vi "Data_Save_GRR.vi"(11 "Data in":T1) -> (1 "Erroe":string[](array[string]), 3 "GRRData":string[](array[string]))   [LabVIEW 2017]
uses:
  Ctrls/CSV_Data.ctl
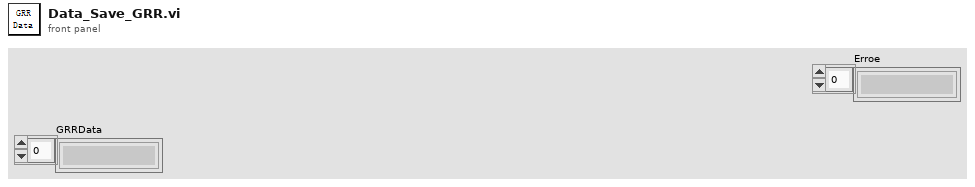
[diagram p1: front panel]
types:
  T1 = typedef "CSV_Data.ctl" = cluster{"Initialisation":cluster{"LMT - Connect UUT (con COM)":string, "LMT - Software Version (rrel)":string, "LMT - Write SKU file (wskuc)":string, "LMT - SKU file name":string, "Connect UUT DDM":string, "Read DDM EOL Timestamp - Mode":string, "Read DDM EOL Timestamp - Timestamp":string, "Read DDM EOL Timestamp - Rig ID":string, "Read DDM EOL Timestamp - Passmark ID":string, "Read DDM EOL Timestamp - Passmark Rev":string, "Software Version before flashing":string, "Read Hardware Serial":string, "UUT DDM SN":string, "Compare DDM SN with MES SN":string, "Backup PCBA Calibration EEPROM Response - CAL":string, "Flash Firmware Version":string, "Check SW Version":string, "Read DDM SW Version after flashing":string, "Set SKU Config":string, "Ready Status":string, "Set Device Mode to EOL":string, "DDM Parameter - Voltage":string, "DDM Parameter - Current":string, "DDM Parameter - Power":string, "DDM Parameter - Speed":string, "DDM Parameter - Pressure":string, "Tester Parameter - Voltage":string, "Tester Parameter - Current":string, "Tester Parameter - Power":string, "Tester Parameter - Ambient Pressure":string, "Tester Parameter - Ambient Temperature":string, "Calculated Parameter - DDM Pressure Corrected":string, "Calculated Parameter - DDM Real Power":string, "Calculated Parameter - Delta V":string}, "BEMF_Calibration":cluster{"Calibration Result - eol_cold_bemf_temp":string, "DDM Ambient Temp":string, "Restriction Plate Diameter":string, "Calibration Result - eol_bemf_mp_cold_coef_a":string, "Calibration Result - eol_bemf_mp_cold_coef_b":string, "Calibration Result - eol_bemf_mp_cold_coef_c":string, "Calibration Result - eol_bemf_lsi_cold_ref_coeffs":string, "Get - Calibration Result - eol_bemf_lsi_speed":string, "Get - Calibration Result - eol_bemf_lsi_integral_0":string, "Calibration Result - eol_bemf_lsi_integral_1":string, "Get - Calibration Result - eol_bemf_lsi_integral_2":string, "Get - Calibration Result - eol_cold_bemf":string, "Get - Calibration Result - eol_cold_bemf_fisf":string, "Finalise Calibration":string, "Compare -Calibration Result - eol_cold_bemf":string, "Compare -Calibration Result - eol_cold_bemf_fisf":string}, "ECO":cluster{"Reset Power Tune":string, "Reset BEMF FISF Calibration":string, "Restriction Plate Diameter":string, "ECO - Stabilisation Time":string, "ECO - DDM Parameter - Voltage":string, "ECO - DDM Parameter - Current":string, "ECO - DDM Parameter - Power":string, "ECO - DDM Parameter - Measured Power":string, "ECO - DDM Parameter - Speed":string, "ECO - DDM Parameter - Pressure":string, "ECO - Tester Parameter - Voltage":string, "ECO - Tester Parameter - Current":string, "ECO - Tester Parameter - Power":string, "ECO - Tester Parameter - Ambient Pressure":string, "ECO - Tester Parameter - Ambient Temperature":string, "ECO - Tester Parameter - Ambient Humidity":string, "ECO - Calculated Parameter - DDM Pressure Corrected":string, "ECO - Calculated Parameter - DDM Real Power":string, "ECO - Calculated Parameter - Delta V":string, "ECO - Calculated Parameter - Flowrate":string, "ECO - Calculated Parameter - Airwatt":string, "ECO - Formula":string, "PT ECO - Power Tune Mode Status":string}, "BOOST":cluster{"Restriction Plate Diameter":string, "BOOST - Stabilisation Time":string, "BOOST - DDM Parameter - Voltage":string, "BOOST - DDM Parameter - Current":string, "BOOST - DDM Parameter - Power":string, "BOOST - DDM Parameter - Measured Power":string, "BOOST - DDM Parameter - Speed":string, "BOOST - DDM Parameter - Pressure":string, "BOOST - Tester Parameter - Voltage":string, "BOOST - Tester Parameter - Current":string, "BOOST - Tester Parameter - Power":string, "BOOST - Tester Parameter - Ambient Pressure":string, "BOOST - Tester Parameter - Ambient Temperature":string, "BOOST - Tester Parameter - Ambient Humidity":string, "BOOST - Calculated Parameter - DDM Pressure Corrected":string, "BOOST - Calculated Parameter - DDM Real Power":string, "BOOST - Calculated Parameter - Delta V":string, "BOOST - Calculated Parameter - Flowrate":string, "BOOST - Calculated Parameter - Airwatt":string, "BOOST - Get AM Presence":string, "Air Muscle Turn Off Status":string, "BOOST - Air Muscle Calculated Parameter - Airwatt B":string, "BOOST - Air Muscle Calculate Airwatt Delta":string, "PT BOOST - Power Tune Mode Status":string, "Finalise Calibration":string, "ECO - Get AW Calibration value":string, "BOOST - Get AW Calibration value":string}, "MAX":cluster{"Restriction Plate Diameter":string, "MAX - Stabilisation Time":string, "Get Average Delta Tmag (LSIdelta_FISFdelta_LSItmag_FISFtmag_IIRtmag)":string, "Get Average Delta Tmag FISF":string, "MAX - DDM Parameter - Voltage":string, "MAX - DDM Parameter - Current":string, "MAX - DDM Parameter - Power":string, "MAX - DDM Parameter - Measured Power":string, "MAX - DDM Parameter - Speed":string, "MAX - DDM Parameter - Pressure":string, "MAX - Tester Parameter - Voltage":string, "MAX - Tester Parameter - Current":string, "MAX - Tester Parameter - Power":string, "MAX - Tester Parameter - Ambient Pressure":string, "MAX - Tester Parameter - Ambient Temperature":string, "MAX - Tester Parameter - Ambient Humidity":string, "MAX - Calculated Parameter - DDM Pressure Corrected":string, "MAX - Calculated Parameter - DDM Real Power":string, "MAX - Calculated Parameter - Delta V":string, "MAX - Calculated Parameter - Flowrate":string, "MAX - Calculated Parameter - Airwatt":string, "MAX_FISF_Check_Average_Delta_Tmag":string, "MAX - FISF - BEMF Finetune Result":string, "MAX tune - Delta P1":string, "MAX tune - Calculated Parameter - Airwatt":string, "Calculate Delta Airwatts - MAX finetune - Delta P2":string, "MAX finetune - DDM Parameter - Voltage":string, "MAX finetune - DDM Parameter - Current":string, "MAX finetune - DDM Parameter - Power":string, "MAX finetune - DDM Parameter - Measured Power":string, "MAX finetune - DDM Parameter - Speed":string, "MAX finetune - DDM Parameter - Pressure":string, "MAX finetune - Tester Parameter - Voltage":string, "MAX finetune - Tester Parameter - Current":string, "MAX finetune - Tester Parameter - Power":string, "MAX finetune - Tester Parameter - Ambient Pressure":string, "MAX finetune - Tester Parameter - Ambient Temperature":string, "MAX finetune - Tester Parameter - Ambient Humidity":string, "MAX finetune - Calculated Parameter - DDM Pressure Corrected":string, "MAX finetune - Calculated Parameter - DDM Real Power":string, "MAX finetune - Calculated Parameter - Delta V":string, "MAX finetune - Calculated Parameter - Flowrate":string, "MAX finetune - Calculated Parameter - Airwatt":string, "Check Derate Result":string, "Delta Tmag FISF":string, "Get Hot BEMF Result":string, "Calculate delta Pressure":string, "Finalise Calibration":string, "Calculate & Check Delta BEMF":string, "Delta P Airwatts Value":string}, "LL":cluster{"DDM Ambient Temp":string, "Restriction Plate Diameter":string, "LL - DDM Parameter - Voltage":string, "LL - DDM Parameter - Current":string, "LL - DDM Parameter - Power":string, "LL - DDM Parameter - Measured Power":string, "LL - DDM Parameter - Speed":string, "LL - DDM Parameter - Pressure":string, "LL - Tester Parameter - Voltage":string, "LL - Tester Parameter - Current":string, "LL - Tester Parameter - Power":string, "LL - DDM Real Power":string, "LL - Calibrate Task Detect LL":string}, "HL":cluster{"HL - DDM Parameter - Voltage":string, "HL - DDM Parameter - Current":string, "HL - DDM Parameter - Power":string, "HL - DDM Parameter - Measured Power":string, "HL - DDM Parameter - Speed":string, "HL - DDM Parameter - Pressure":string, "HL - Tester Parameter - Voltage":string, "HL - Tester Parameter - Current":string, "HL - Tester Parameter - Power":string, "HL - DDM Real Power":string, "HL - Calibrate Task Detect HL":string}, "LH":cluster{"Restriction Plate Diameter":string, "LH - DDM Parameter - Voltage":string, "LH - DDM Parameter - Current":string, "LH - DDM Parameter - Power":string, "LH - DDM Parameter - Measured Power":string, "LH - DDM Parameter - Speed":string, "LH - DDM Parameter - Pressure":string, "LH - Tester Parameter - Voltage":string, "LH - Tester Parameter - Current":string, "LH - Tester Parameter - Power":string, "LH - DDM Real Power":string, "LH - Calibrate Task Detect LH":string}, "HH":cluster{"HH - DDM Parameter - Voltage":string, "HH - DDM Parameter - Current":string, "HH - DDM Parameter - Power":string, "HH - DDM Parameter - Measured Power":string, "HH - DDM Parameter - Speed":string, "HH - DDM Parameter - Pressure":string, "HH - Tester Parameter - Voltage":string, "HH - Tester Parameter - Current":string, "HH - Tester Parameter - Power":string, "HH - DDM Real Power":string, "HH - Calibrate Task Detect HH":string}, "Inlet Blockage Calibration":cluster{"Inlet Blockage Calibration - DDM Parameter - Voltage":string, "Inlet Blockage Calibration - DDM Parameter - Current":string, "Inlet Blockage Calibration - DDM Parameter - Power":string, "Inlet Blockage Calibration - DDM Parameter - Measured Power":string, "Inlet Blockage Calibration - DDM Parameter - Speed":string, "Inlet Blockage Calibration - DDM Parameter - Pressure":string, "Inlet Blockage Calibration - Tester Parameter - Voltage":string, "Inlet Blockage Calibration - Tester Parameter - Current":string, "Inlet Blockage Calibration - Tester Parameter - Power":string, "Inlet Blockage Calibration - DDM Real Power":string, "Calibration Inlet Blockage_E":string, "Finalise Calibration":string, "Get Task Detect LL":string, "Get Task Detect HL":string, "Get Task Detect LH":string, "Get Task Detect HH":string, "Calibration Inlet Blockage":string, "Calibration eol cold bemf temp":string}, "GOOD":cluster{"GOOD UNIT - Clear EEPROM Error Log":string, "GOOD UNIT - Write Product Timestamp - Mode":string, "GOOD UNIT - Write Product Timestamp - Timestamp":string, "GOOD UNIT - Write Product Timestamp - Rig ID":string, "GOOD UNIT - Write Product Timestamp - Passmark ID":string, "GOOD UNIT - Write Product Timestamp - Passmark Rev":string, "GOOD UNIT - Set Device Mode to PROD":string, "GOOD UNIT - Backup PCBA Calibration EEPROM Response":string, "GOOD UNIT - Check Security Bit":string, "GOOD UNIT - Set Calibration Lock":string, "GOOD UNIT - Get_Calibration_Lock":string, "GOOD UNIT - Disconnect UUT":string}, "NG":cluster{"NG UNIT - Read NVM Error":string, "NG UNIT - Set Device Mode to FCT":string, "NG UNIT - Backup PCBA Calibration EEPROM Response - CAL":string, "NG UNIT - Backup PCBA Calibration EEPROM Response - ERROR":string, "NG UNIT - Backup PCBA Calibration EEPROM Response - USAGE":string, "NG UNIT - Disconnect UUT":string}, "SN":string, "Table":string[][], "Count":cluster{"Total":i32, "OK":i32, "NG":i32, "Yield":dbl}, "Start Time":timestamp, "daemon reference":refnum<k5>, "CT":dbl, "Config":string[][], "OK/NG":bool, "Station ID":string, "MES DDM SN":string, "MES PCBA SN":string, "Retest":string, "UID":string, "Initialisation_Status":cluster{"LMT - Connect UUT (con COM)":string, "LMT - Software Version (rrel)":string, "LMT - Write SKU file (wskuc)":string, "LMT - SKU file name":string, "Connect UUT DDM":string, "Read DDM EOL Timestamp - Mode":string, "Read DDM EOL Timestamp - Timestamp":string, "Read DDM EOL Timestamp - Rig ID":string, "Read DDM EOL Timestamp - Passmark ID":string, "Read DDM EOL Timestamp - Passmark Rev":string, "Software Version before flashing":string, "Read Hardware Serial":string, "UUT DDM SN":string, "Compare DDM SN with MES SN":string, "Backup PCBA Calibration EEPROM Response - CAL":string, "Flash Firmware Version":string, "Check SW Version":string, "Read DDM SW Version after flashing":string, "Set SKU Config":string, "Ready Status":string, "Set Device Mode to EOL":string, "DDM Parameter - Voltage":string, "DDM Parameter - Current":string, "DDM Parameter - Power":string, "DDM Parameter - Speed":string, "DDM Parameter - Pressure":string, "Tester Parameter - Voltage":string, "Tester Parameter - Current":string, "Tester Parameter - Power":string, "Tester Parameter - Ambient Pressure":string, "Tester Parameter - Ambient Temperature":string, "Calculated Parameter - DDM Pressure Corrected":string, "Calculated Parameter - DDM Real Power":string, "Calculated Parameter - Delta V":string}, "BEMF_Calibration_Status":cluster{"Calibration Result - eol_cold_bemf_temp":string, "DDM Ambient Temp":string, "Restriction Plate Diameter":string, "Calibration Result - eol_bemf_mp_cold_coef_a":string, "Calibration Result - eol_bemf_mp_cold_coef_b":string, "Calibration Result - eol_bemf_mp_cold_coef_c":string, "Calibration Result - eol_bemf_lsi_cold_ref_coeffs":string, "Get - Calibration Result - eol_bemf_lsi_speed":string, "Get - Calibration Result - eol_bemf_lsi_integral_0":string, "Calibration Result - eol_bemf_lsi_integral_1":string, "Get - Calibration Result - eol_bemf_lsi_integral_2":string, "Get - Calibration Result - eol_cold_bemf":string, "Get - Calibration Result - eol_cold_bemf_fisf":string, "Finalise Calibration":string, "Compare -Calibration Result - eol_cold_bemf":string, "Compare -Calibration Result - eol_cold_bemf_fisf":string}, "ECO_Status":cluster{"Reset Power Tune":string, "Reset BEMF FISF Calibration":string, "Restriction Plate Diameter":string, "ECO - Stabilisation Time":string, "ECO - DDM Parameter - Voltage":string, "ECO - DDM Parameter - Current":string, "ECO - DDM Parameter - Power":string, "ECO - DDM Parameter - Measured Power":string, "ECO - DDM Parameter - Speed":string, "ECO - DDM Parameter - Pressure":string, "ECO - Tester Parameter - Voltage":string, "ECO - Tester Parameter - Current":string, "ECO - Tester Parameter - Power":string, "ECO - Tester Parameter - Ambient Pressure":string, "ECO - Tester Parameter - Ambient Temperature":string, "ECO - Tester Parameter - Ambient Humidity":string, "ECO - Calculated Parameter - DDM Pressure Corrected":string, "ECO - Calculated Parameter - DDM Real Power":string, "ECO - Calculated Parameter - Delta V":string, "ECO - Calculated Parameter - Flowrate":string, "ECO - Calculated Parameter - Airwatt":string, "ECO - Formula":string, "PT ECO - Power Tune Mode Status":string}, "BOOST_Status":cluster{"Restriction Plate Diameter":string, "BOOST - Stabilisation Time":string, "BOOST - DDM Parameter - Voltage":string, "BOOST - DDM Parameter - Current":string, "BOOST - DDM Parameter - Power":string, "BOOST - DDM Parameter - Measured Power":string, "BOOST - DDM Parameter - Speed":string, "BOOST - DDM Parameter - Pressure":string, "BOOST - Tester Parameter - Voltage":string, "BOOST - Tester Parameter - Current":string, "BOOST - Tester Parameter - Power":string, "BOOST - Tester Parameter - Ambient Pressure":string, "BOOST - Tester Parameter - Ambient Temperature":string, "BOOST - Tester Parameter - Ambient Humidity":string, "BOOST - Calculated Parameter - DDM Pressure Corrected":string, "BOOST - Calculated Parameter - DDM Real Power":string, "BOOST - Calculated Parameter - Delta V":string, "BOOST - Calculated Parameter - Flowrate":string, "BOOST - Calculated Parameter - Airwatt":string, "BOOST - Get AM Presence":string, "Air Muscle Turn Off Status":string, "BOOST - Air Muscle Calculated Parameter - Airwatt B":string, "BOOST - Air Muscle Calculate Airwatt Delta":string, "PT BOOST - Power Tune Mode Status":string, "Finalise Calibration":string, "ECO - Get AW Calibration value":string, "BOOST - Get AW Calibration value":string}, "MAX_Status":cluster{"Restriction Plate Diameter":string, "MAX - Stabilisation Time":string, "Get Average Delta Tmag (LSIdelta_FISFdelta_LSItmag_FISFtmag_IIRtmag)":string, "Get Average Delta Tmag FISF":string, "MAX - DDM Parameter - Voltage":string, "MAX - DDM Parameter - Current":string, "MAX - DDM Parameter - Power":string, "MAX - DDM Parameter - Measured Power":string, "MAX - DDM Parameter - Speed":string, "MAX - DDM Parameter - Pressure":string, "MAX - Tester Parameter - Voltage":string, "MAX - Tester Parameter - Current":string, "MAX - Tester Parameter - Power":string, "MAX - Tester Parameter - Ambient Pressure":string, "MAX - Tester Parameter - Ambient Temperature":string, "MAX - Tester Parameter - Ambient Humidity":string, "MAX - Calculated Parameter - DDM Pressure Corrected":string, "MAX - Calculated Parameter - DDM Real Power":string, "MAX - Calculated Parameter - Delta V":string, "MAX - Calculated Parameter - Flowrate":string, "MAX - Calculated Parameter - Airwatt":string, "MAX_FISF_Check_Average_Delta_Tmag":string, "MAX - FISF - BEMF Finetune Result":string, "MAX tune - Delta P1":string, "MAX tune - Calculated Parameter - Airwatt":string, "Calculate Delta Airwatts - MAX finetune - Delta P2":string, "MAX finetune - DDM Parameter - Voltage":string, "MAX finetune - DDM Parameter - Current":string, "MAX finetune - DDM Parameter - Power":string, "MAX finetune - DDM Parameter - Measured Power":string, "MAX finetune - DDM Parameter - Speed":string, "MAX finetune - DDM Parameter - Pressure":string, "MAX finetune - Tester Parameter - Voltage":string, "MAX finetune - Tester Parameter - Current":string, "MAX finetune - Tester Parameter - Power":string, "MAX finetune - Tester Parameter - Ambient Pressure":string, "MAX finetune - Tester Parameter - Ambient Temperature":string, "MAX finetune - Tester Parameter - Ambient Humidity":string, "MAX finetune - Calculated Parameter - DDM Pressure Corrected":string, "MAX finetune - Calculated Parameter - DDM Real Power":string, "MAX finetune - Calculated Parameter - Delta V":string, "MAX finetune - Calculated Parameter - Flowrate":string, "MAX finetune - Calculated Parameter - Airwatt":string, "Check Derate Result":string, "Delta Tmag FISF":string, "Get Hot BEMF Result":string, "Calculate delta Pressure":string, "Finalise Calibration":string, "Calculate & Check Delta BEMF":string, "Delta P Airwatts Value":string}, "LL_Status":cluster{"DDM Ambient Temp":string, "Restriction Plate Diameter":string, "LL - DDM Parameter - Voltage":string, "LL - DDM Parameter - Current":string, "LL - DDM Parameter - Power":string, "LL - DDM Parameter - Measured Power":string, "LL - DDM Parameter - Speed":string, "LL - DDM Parameter - Pressure":string, "LL - Tester Parameter - Voltage":string, "LL - Tester Parameter - Current":string, "LL - Tester Parameter - Power":string, "LL - DDM Real Power":string, "LL - Calibrate Task Detect LL":string}, "HL_Status":cluster{"HL - DDM Parameter - Voltage":string, "HL - DDM Parameter - Current":string, "HL - DDM Parameter - Power":string, "HL - DDM Parameter - Measured Power":string, "HL - DDM Parameter - Speed":string, "HL - DDM Parameter - Pressure":string, "HL - Tester Parameter - Voltage":string, "HL - Tester Parameter - Current":string, "HL - Tester Parameter - Power":string, "HL - DDM Real Power":string, "HL - Calibrate Task Detect HL":string}, "LH_Status":cluster{"Restriction Plate Diameter":string, "LH - DDM Parameter - Voltage":string, "LH - DDM Parameter - Current":string, "LH - DDM Parameter - Power":string, "LH - DDM Parameter - Measured Power":string, "LH - DDM Parameter - Speed":string, "LH - DDM Parameter - Pressure":string, "LH - Tester Parameter - Voltage":string, "LH - Tester Parameter - Current":string, "LH - Tester Parameter - Power":string, "LH - DDM Real Power":string, "LH - Calibrate Task Detect LH":string}, "HH_Status":cluster{"HH - DDM Parameter - Voltage":string, "HH - DDM Parameter - Current":string, "HH - DDM Parameter - Power":string, "HH - DDM Parameter - Measured Power":string, "HH - DDM Parameter - Speed":string, "HH - DDM Parameter - Pressure":string, "HH - Tester Parameter - Voltage":string, "HH - Tester Parameter - Current":string, "HH - Tester Parameter - Power":string, "HH - DDM Real Power":string, "HH - Calibrate Task Detect HH":string}, "Inlet Blockage Calibration_Status":cluster{"Inlet Blockage Calibration - DDM Parameter - Voltage":string, "Inlet Blockage Calibration - DDM Parameter - Current":string, "Inlet Blockage Calibration - DDM Parameter - Power":string, "Inlet Blockage Calibration - DDM Parameter - Measured Power":string, "Inlet Blockage Calibration - DDM Parameter - Speed":string, "Inlet Blockage Calibration - DDM Parameter - Pressure":string, "Inlet Blockage Calibration - Tester Parameter - Voltage":string, "Inlet Blockage Calibration - Tester Parameter - Current":string, "Inlet Blockage Calibration - Tester Parameter - Power":string, "Inlet Blockage Calibration - DDM Real Power":string, "Calibration Inlet Blockage_E":string, "Finalise Calibration":string, "Get Task Detect LL":string, "Get Task Detect HL":string, "Get Task Detect LH":string, "Get Task Detect HH":string, "Calibration Inlet Blockage":string, "Calibration eol cold bemf temp":string}, "GOOD_Status":cluster{"GOOD UNIT - Clear EEPROM Error Log":string, "GOOD UNIT - Write Product Timestamp - Mode":string, "GOOD UNIT - Write Product Timestamp - Timestamp":string, "GOOD UNIT - Write Product Timestamp - Rig ID":string, "GOOD UNIT - Write Product Timestamp - Passmark ID":string, "GOOD UNIT - Write Product Timestamp - Passmark Rev":string, "GOOD UNIT - Set Device Mode to PROD":string, "GOOD UNIT - Backup PCBA Calibration EEPROM Response":string, "GOOD UNIT - Check Security Bit":string, "GOOD UNIT - Set Calibration Lock":string, "GOOD UNIT - Get_Calibration_Lock":string, "GOOD UNIT - Disconnect UUT":string}, "NG_Status":cluster{"NG UNIT - Read NVM Error":string, "NG UNIT - Set Device Mode to FCT":string, "NG UNIT - Backup PCBA Calibration EEPROM Response - CAL":string, "NG UNIT - Backup PCBA Calibration EEPROM Response - ERROR":string, "NG UNIT - Backup PCBA Calibration EEPROM Response - USAGE":string, "NG UNIT - Disconnect UUT":string}, "SKU":string, "Plate_Diameter":string, "Alarm":string}
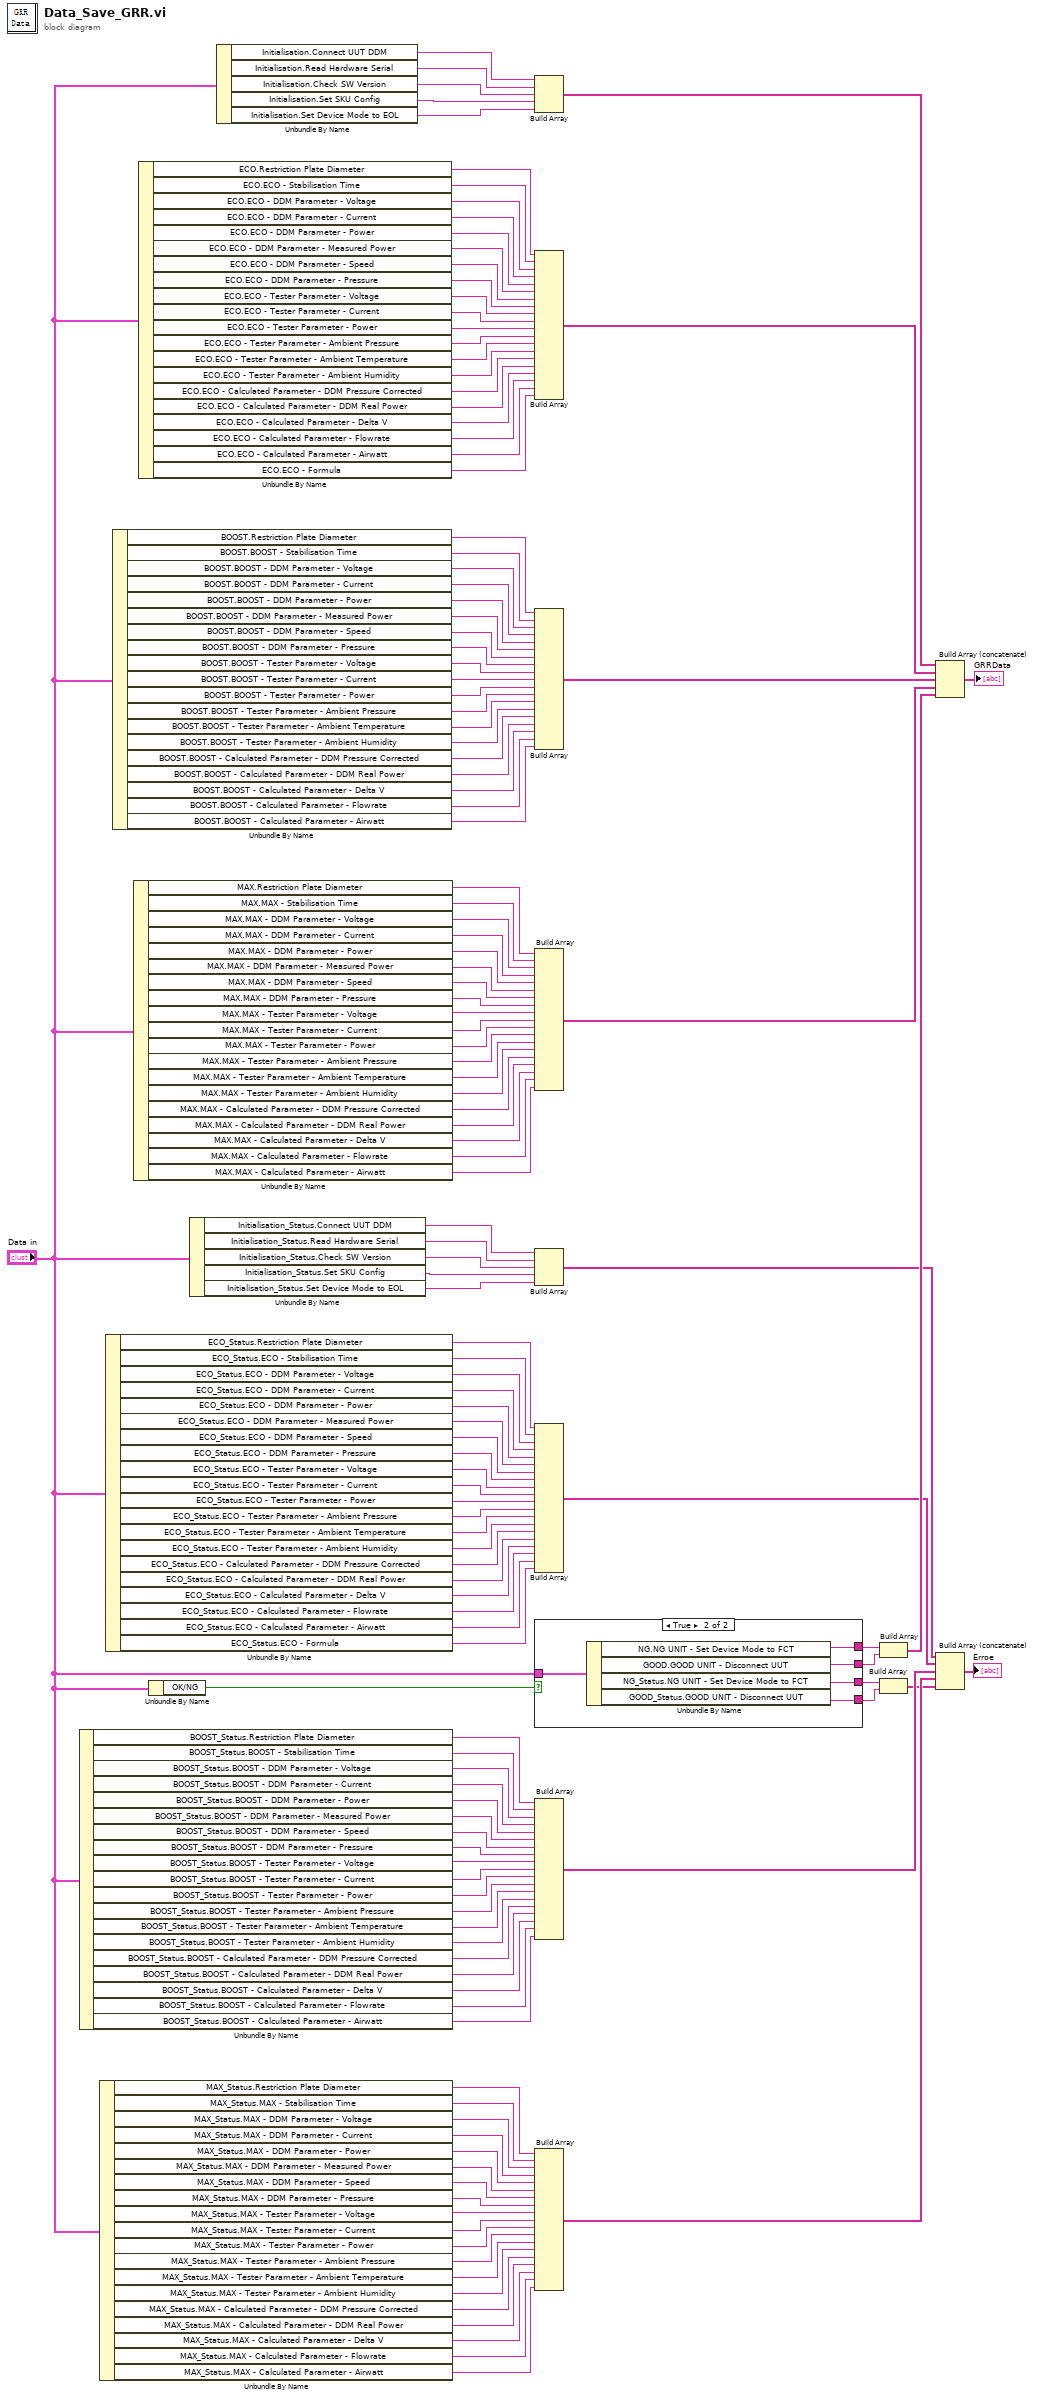
[diagram p0: block diagram]
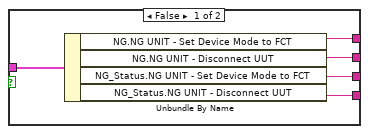
[diagram p2: hidden frame]
diagram:
  n1 = Unbundle By Name("Data in") -> ("BOOST_Status.Restriction Plate Diameter"=w46:string, "BOOST_Status.BOOST - Stabilisation Time"=w45:string, "BOOST_Status.BOOST - DDM Parameter - Voltage"=w44:string, "BOOST_Status.BOOST - DDM Parameter - Current"=w43:string, "BOOST_Status.BOOST - DDM Parameter - Power"=w42:string, "BOOST_Status.BOOST - DDM Parameter - Measured Power"=w41:string, "BOOST_Status.BOOST - DDM Parameter - Speed"=w40:string, "BOOST_Status.BOOST - DDM Parameter - Pressure"=w39:string, "BOOST_Status.BOOST - Tester Parameter - Voltage"=w38:string, "BOOST_Status.BOOST - Tester Parameter - Current"=w37:string, "BOOST_Status.BOOST - Tester Parameter - Power"=w36:string, "BOOST_Status.BOOST - Tester Parameter - Ambient Pressure"=w35:string, "BOOST_Status.BOOST - Tester Parameter - Ambient Temperature"=w34:string, "BOOST_Status.BOOST - Tester Parameter - Ambient Humidity"=w33:string, "BOOST_Status.BOOST - Calculated Parameter - DDM Pressure Corrected"=w32:string, "BOOST_Status.BOOST - Calculated Parameter - DDM Real Power"=w31:string, "BOOST_Status.BOOST - Calculated Parameter - Delta V"=w30:string, "BOOST_Status.BOOST - Calculated Parameter - Flowrate"=w29:string, "BOOST_Status.BOOST - Calculated Parameter - Airwatt"=w28:string)
  n2 = Unbundle By Name("Data in") -> ("MAX_Status.Restriction Plate Diameter"=w27:string, "MAX_Status.MAX - Stabilisation Time"=w26:string, "MAX_Status.MAX - DDM Parameter - Voltage"=w25:string, "MAX_Status.MAX - DDM Parameter - Current"=w24:string, "MAX_Status.MAX - DDM Parameter - Power"=w23:string, "MAX_Status.MAX - DDM Parameter - Measured Power"=w22:string, "MAX_Status.MAX - DDM Parameter - Speed"=w21:string, "MAX_Status.MAX - DDM Parameter - Pressure"=w20:string, "MAX_Status.MAX - Tester Parameter - Voltage"=w19:string, "MAX_Status.MAX - Tester Parameter - Current"=w18:string, "MAX_Status.MAX - Tester Parameter - Power"=w17:string, "MAX_Status.MAX - Tester Parameter - Ambient Pressure"=w16:string, "MAX_Status.MAX - Tester Parameter - Ambient Temperature"=w15:string, "MAX_Status.MAX - Tester Parameter - Ambient Humidity"=w14:string, "MAX_Status.MAX - Calculated Parameter - DDM Pressure Corrected"=w13:string, "MAX_Status.MAX - Calculated Parameter - DDM Real Power"=w12:string, "MAX_Status.MAX - Calculated Parameter - Delta V"=w11:string, "MAX_Status.MAX - Calculated Parameter - Flowrate"=w10:string, "MAX_Status.MAX - Calculated Parameter - Airwatt"=w9:string)
  n3 = Unbundle By Name("Data in") -> ("ECO_Status.Restriction Plate Diameter"=w66:string, "ECO_Status.ECO - Stabilisation Time"=w65:string, "ECO_Status.ECO - DDM Parameter - Voltage"=w64:string, "ECO_Status.ECO - DDM Parameter - Current"=w63:string, "ECO_Status.ECO - DDM Parameter - Power"=w62:string, "ECO_Status.ECO - DDM Parameter - Measured Power"=w61:string, "ECO_Status.ECO - DDM Parameter - Speed"=w60:string, "ECO_Status.ECO - DDM Parameter - Pressure"=w59:string, "ECO_Status.ECO - Tester Parameter - Voltage"=w58:string, "ECO_Status.ECO - Tester Parameter - Current"=w57:string, "ECO_Status.ECO - Tester Parameter - Power"=w56:string, "ECO_Status.ECO - Tester Parameter - Ambient Pressure"=w55:string, "ECO_Status.ECO - Tester Parameter - Ambient Temperature"=w54:string, "ECO_Status.ECO - Tester Parameter - Ambient Humidity"=w53:string, "ECO_Status.ECO - Calculated Parameter - DDM Pressure Corrected"=w52:string, "ECO_Status.ECO - Calculated Parameter - DDM Real Power"=w51:string, "ECO_Status.ECO - Calculated Parameter - Delta V"=w50:string, "ECO_Status.ECO - Calculated Parameter - Flowrate"=w49:string, "ECO_Status.ECO - Calculated Parameter - Airwatt"=w48:string, "ECO_Status.ECO - Formula"=w47:string)
  n4 = Unbundle By Name("Data in") -> ("BOOST.Restriction Plate Diameter"=w117:string, "BOOST.BOOST - Stabilisation Time"=w116:string, "BOOST.BOOST - DDM Parameter - Voltage"=w115:string, "BOOST.BOOST - DDM Parameter - Current"=w114:string, "BOOST.BOOST - DDM Parameter - Power"=w113:string, "BOOST.BOOST - DDM Parameter - Measured Power"=w112:string, "BOOST.BOOST - DDM Parameter - Speed"=w111:string, "BOOST.BOOST - DDM Parameter - Pressure"=w110:string, "BOOST.BOOST - Tester Parameter - Voltage"=w109:string, "BOOST.BOOST - Tester Parameter - Current"=w108:string, "BOOST.BOOST - Tester Parameter - Power"=w107:string, "BOOST.BOOST - Tester Parameter - Ambient Pressure"=w106:string, "BOOST.BOOST - Tester Parameter - Ambient Temperature"=w105:string, "BOOST.BOOST - Tester Parameter - Ambient Humidity"=w104:string, "BOOST.BOOST - Calculated Parameter - DDM Pressure Corrected"=w103:string, "BOOST.BOOST - Calculated Parameter - DDM Real Power"=w102:string, "BOOST.BOOST - Calculated Parameter - Delta V"=w101:string, "BOOST.BOOST - Calculated Parameter - Flowrate"=w100:string, "BOOST.BOOST - Calculated Parameter - Airwatt"=w99:string)
  n5 = Unbundle By Name("Data in") -> ("MAX.Restriction Plate Diameter"=w98:string, "MAX.MAX - Stabilisation Time"=w97:string, "MAX.MAX - DDM Parameter - Voltage"=w96:string, "MAX.MAX - DDM Parameter - Current"=w95:string, "MAX.MAX - DDM Parameter - Power"=w94:string, "MAX.MAX - DDM Parameter - Measured Power"=w93:string, "MAX.MAX - DDM Parameter - Speed"=w92:string, "MAX.MAX - DDM Parameter - Pressure"=w91:string, "MAX.MAX - Tester Parameter - Voltage"=w90:string, "MAX.MAX - Tester Parameter - Current"=w89:string, "MAX.MAX - Tester Parameter - Power"=w88:string, "MAX.MAX - Tester Parameter - Ambient Pressure"=w87:string, "MAX.MAX - Tester Parameter - Ambient Temperature"=w86:string, "MAX.MAX - Tester Parameter - Ambient Humidity"=w85:string, "MAX.MAX - Calculated Parameter - DDM Pressure Corrected"=w84:string, "MAX.MAX - Calculated Parameter - DDM Real Power"=w83:string, "MAX.MAX - Calculated Parameter - Delta V"=w82:string, "MAX.MAX - Calculated Parameter - Flowrate"=w81:string, "MAX.MAX - Calculated Parameter - Airwatt"=w80:string)
  n6 = Unbundle By Name("Data in") -> ("ECO.Restriction Plate Diameter"=w135:string, "ECO.ECO - Stabilisation Time"=w137:string, "ECO.ECO - DDM Parameter - Voltage"=w136:string, "ECO.ECO - DDM Parameter - Current"=w134:string, "ECO.ECO - DDM Parameter - Power"=w133:string, "ECO.ECO - DDM Parameter - Measured Power"=w132:string, "ECO.ECO - DDM Parameter - Speed"=w131:string, "ECO.ECO - DDM Parameter - Pressure"=w130:string, "ECO.ECO - Tester Parameter - Voltage"=w129:string, "ECO.ECO - Tester Parameter - Current"=w128:string, "ECO.ECO - Tester Parameter - Power"=w127:string, "ECO.ECO - Tester Parameter - Ambient Pressure"=w126:string, "ECO.ECO - Tester Parameter - Ambient Temperature"=w125:string, "ECO.ECO - Tester Parameter - Ambient Humidity"=w124:string, "ECO.ECO - Calculated Parameter - DDM Pressure Corrected"=w123:string, "ECO.ECO - Calculated Parameter - DDM Real Power"=w122:string, "ECO.ECO - Calculated Parameter - Delta V"=w121:string, "ECO.ECO - Calculated Parameter - Flowrate"=w120:string, "ECO.ECO - Calculated Parameter - Airwatt"=w119:string, "ECO.ECO - Formula"=w118:string)
  n7 = Unbundle By Name("Data in") -> ("OK/NG"=w138:bool)
  n8 = Unbundle By Name("Data in") -> ("Initialisation_Status.Connect UUT DDM"=w72:string, "Initialisation_Status.Read Hardware Serial"=w71:string, "Initialisation_Status.Check SW Version"=w70:string, "Initialisation_Status.Set SKU Config"=w69:string, "Initialisation_Status.Set Device Mode to EOL"=w68:string)
  n9 = Unbundle By Name("Data in") -> ("Initialisation.Connect UUT DDM"=w144:string, "Initialisation.Read Hardware Serial"=w143:string, "Initialisation.Check SW Version"=w142:string, "Initialisation.Set SKU Config"=w141:string, "Initialisation.Set Device Mode to EOL"=w140:string)
  n10 = Build Array(w144, w143, w142, w141, w140) -> (w139:string[])
  n11 = Build Array(w135, w137, w136, w134, w133, w132, w131, w130, w129, w128, w127, w126, w125, w124, w123, w122, w121, w120, w119, w118) -> (w79:string[])
  n12 = Build Array(w117, w116, w115, w114, w113, w112, w111, w110, w109, w108, w107, w106, w105, w104, w103, w102, w101, w100, w99) -> (w78:string[])
  n13 = Build Array(w98, w97, w96, w95, w94, w93, w92, w91, w90, w89, w88, w87, w86, w85, w84, w83, w82, w81, w80) -> (w77:string[])
  n14 = Build Array(w72, w71, w70, w69, w68) -> (w6:string[])
  n15 = Build Array(w66, w65, w64, w63, w62, w61, w60, w59, w58, w57, w56, w55, w54, w53, w52, w51, w50, w49, w48, w47) -> (w5:string[])
  n16 = case shown="True" w138 {
    tunnel: "Data in" -> [w149 w154]
    tunnel: [w148 w153] -> w75
    tunnel: [w147 w152] -> w76
    tunnel: [w146 w151] -> w8
    tunnel: [w145 w150] -> w7
    frame False {
      n17 = Unbundle By Name(w149) -> ("NG.NG UNIT - Set Device Mode to FCT"=w148:string, "NG.NG UNIT - Disconnect UUT"=w147:string, "NG_Status.NG UNIT - Set Device Mode to FCT"=w146:string, "NG_Status.NG UNIT - Disconnect UUT"=w145:string)
    }
    frame True {
      n18 = Unbundle By Name(w154) -> ("NG.NG UNIT - Set Device Mode to FCT"=w153:string, "GOOD.GOOD UNIT - Disconnect UUT"=w152:string, "NG_Status.NG UNIT - Set Device Mode to FCT"=w151:string, "GOOD_Status.GOOD UNIT - Disconnect UUT"=w150:string)
    }
  }
  n19 = Build Array(w46, w45, w44, w43, w42, w41, w40, w39, w38, w37, w36, w35, w34, w33, w32, w31, w30, w29, w28) -> (w4:string[])
  n20 = Build Array(w27, w26, w25, w24, w23, w22, w21, w20, w19, w18, w17, w16, w15, w14, w13, w12, w11, w10, w9) -> (w3:string[])
  n21 = Build Array(w75, w76) -> (w74:string[])
  n22 = Build Array(w8, w7) -> (w2:string[])
  n23 = Build Array (concatenate)(w139, w79, w78, w77, w74) -> (→"GRRData":string[])
  n24 = Build Array (concatenate)(w6, w5, w4, w3, w2) -> (→"Erroe":string[])
